vi "Read timeouts.vi"(8 "error in (no error)":errorcluster, 11 "Server in":refnum<class "TCP-Server.lvclass">) -> (0 "error out":errorcluster, 1 "ms create listener":i32=2000, 2 "ms timeout listening":i32, 3 "Server out":refnum<class "TCP-Server.lvclass">, 4 "ms rec message":i32, 6 "ms send status":i32)   [LabVIEW 2018, in "TCP-Server.lvclass"]
uses:
  TCP-Server.lvclass
  TCP-Server.lvclass/TCP-Server.ctl
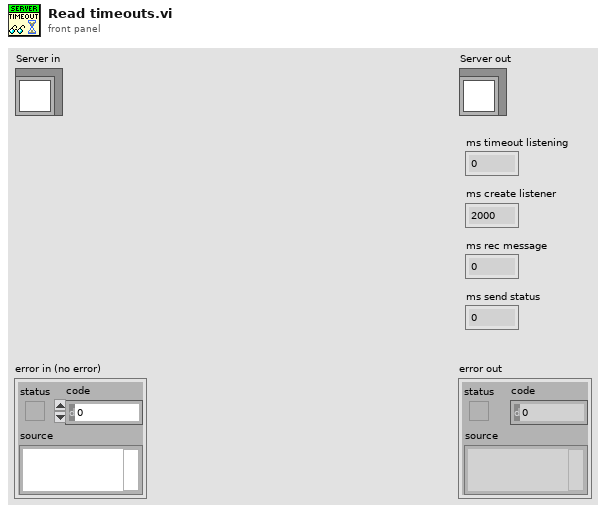
[diagram p1: front panel]
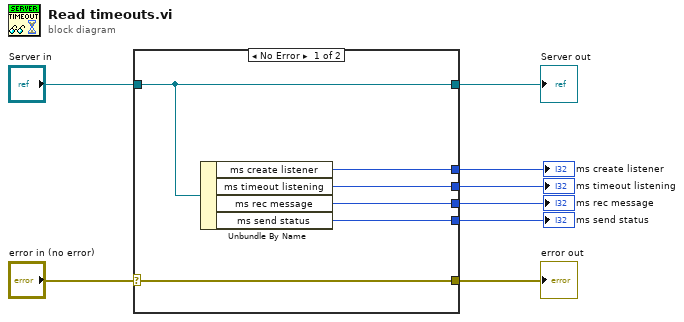
[diagram p0: block diagram]
diagram:
  n1 = case shown="No Error" "error in (no error)" {
    selector: "error in (no error)" -> [w14 w15]
    tunnel: [w14 w15] -> w7
    tunnel: [w13 w16] -> w5
    tunnel: "Server in" -> [w13 w16]
    tunnel: [w12 _] -> w4
    tunnel: [w11 _] -> w3
    tunnel: [w10 _] -> w2
    tunnel: [w9 _] -> w1
    frame No Error {
      n2 = Unbundle By Name(w13) -> ("ms create listener"=w12:i32, "ms timeout listening"=w10:i32, "ms rec message"=w9:i32, "ms send status"=w11:i32)
    }
    frame Error {
    }
  }
  "error out" <- w7
  "Server out" <- w5
  "ms create listener" <- w4
  "ms send status" <- w3
  "ms timeout listening" <- w2
  "ms rec message" <- w1
